vi "Generate_WayPoints_Hopping_CV_VUW.vi"(8 "NumberOfCVsAtEachPoint":i32=1, 11 "Input Cluster":T2={"Scan Rate (um/s)"=15.0, "X Start"=15.0, "X End"=15.0, "Y Start"=15.0, "Y End"=15.0, " Z Start"=15.0, "HoppingDistance"=1.0, "V"=15.0, "Z End"=15.0, "Approach Rate Hopping (um/s)"=15.0, "Retrack Rate (um/s)"=15.0, "V 2"=15.0, "Approach Rate (um/s)"=15.0, "V 3"=15.0, "CV Rate / V/s"=15.0, "V 4"=15.0, "V 1"=15.0, "HoldTime1/s"=15.0, "Hold time 2 / s"=15.0, "Hold time 3/ s"=15.0, "HoppingDistanceBetweenLines"=1.0}) -> (0 "output cluster":T1, 3 "WaitTimeScaler":u64)   [LabVIEW 2023]
uses:
  TypeDefs/WayPointCluster.ctl
  TypeDefsControls/Time.ctl
  User_Vi/Settings.vi
panel:
  in  "WayPointCluster 2":T1
  out "Y  P":dbl
  out "X  P":dbl
  out "HoppingDistanceX":dbl
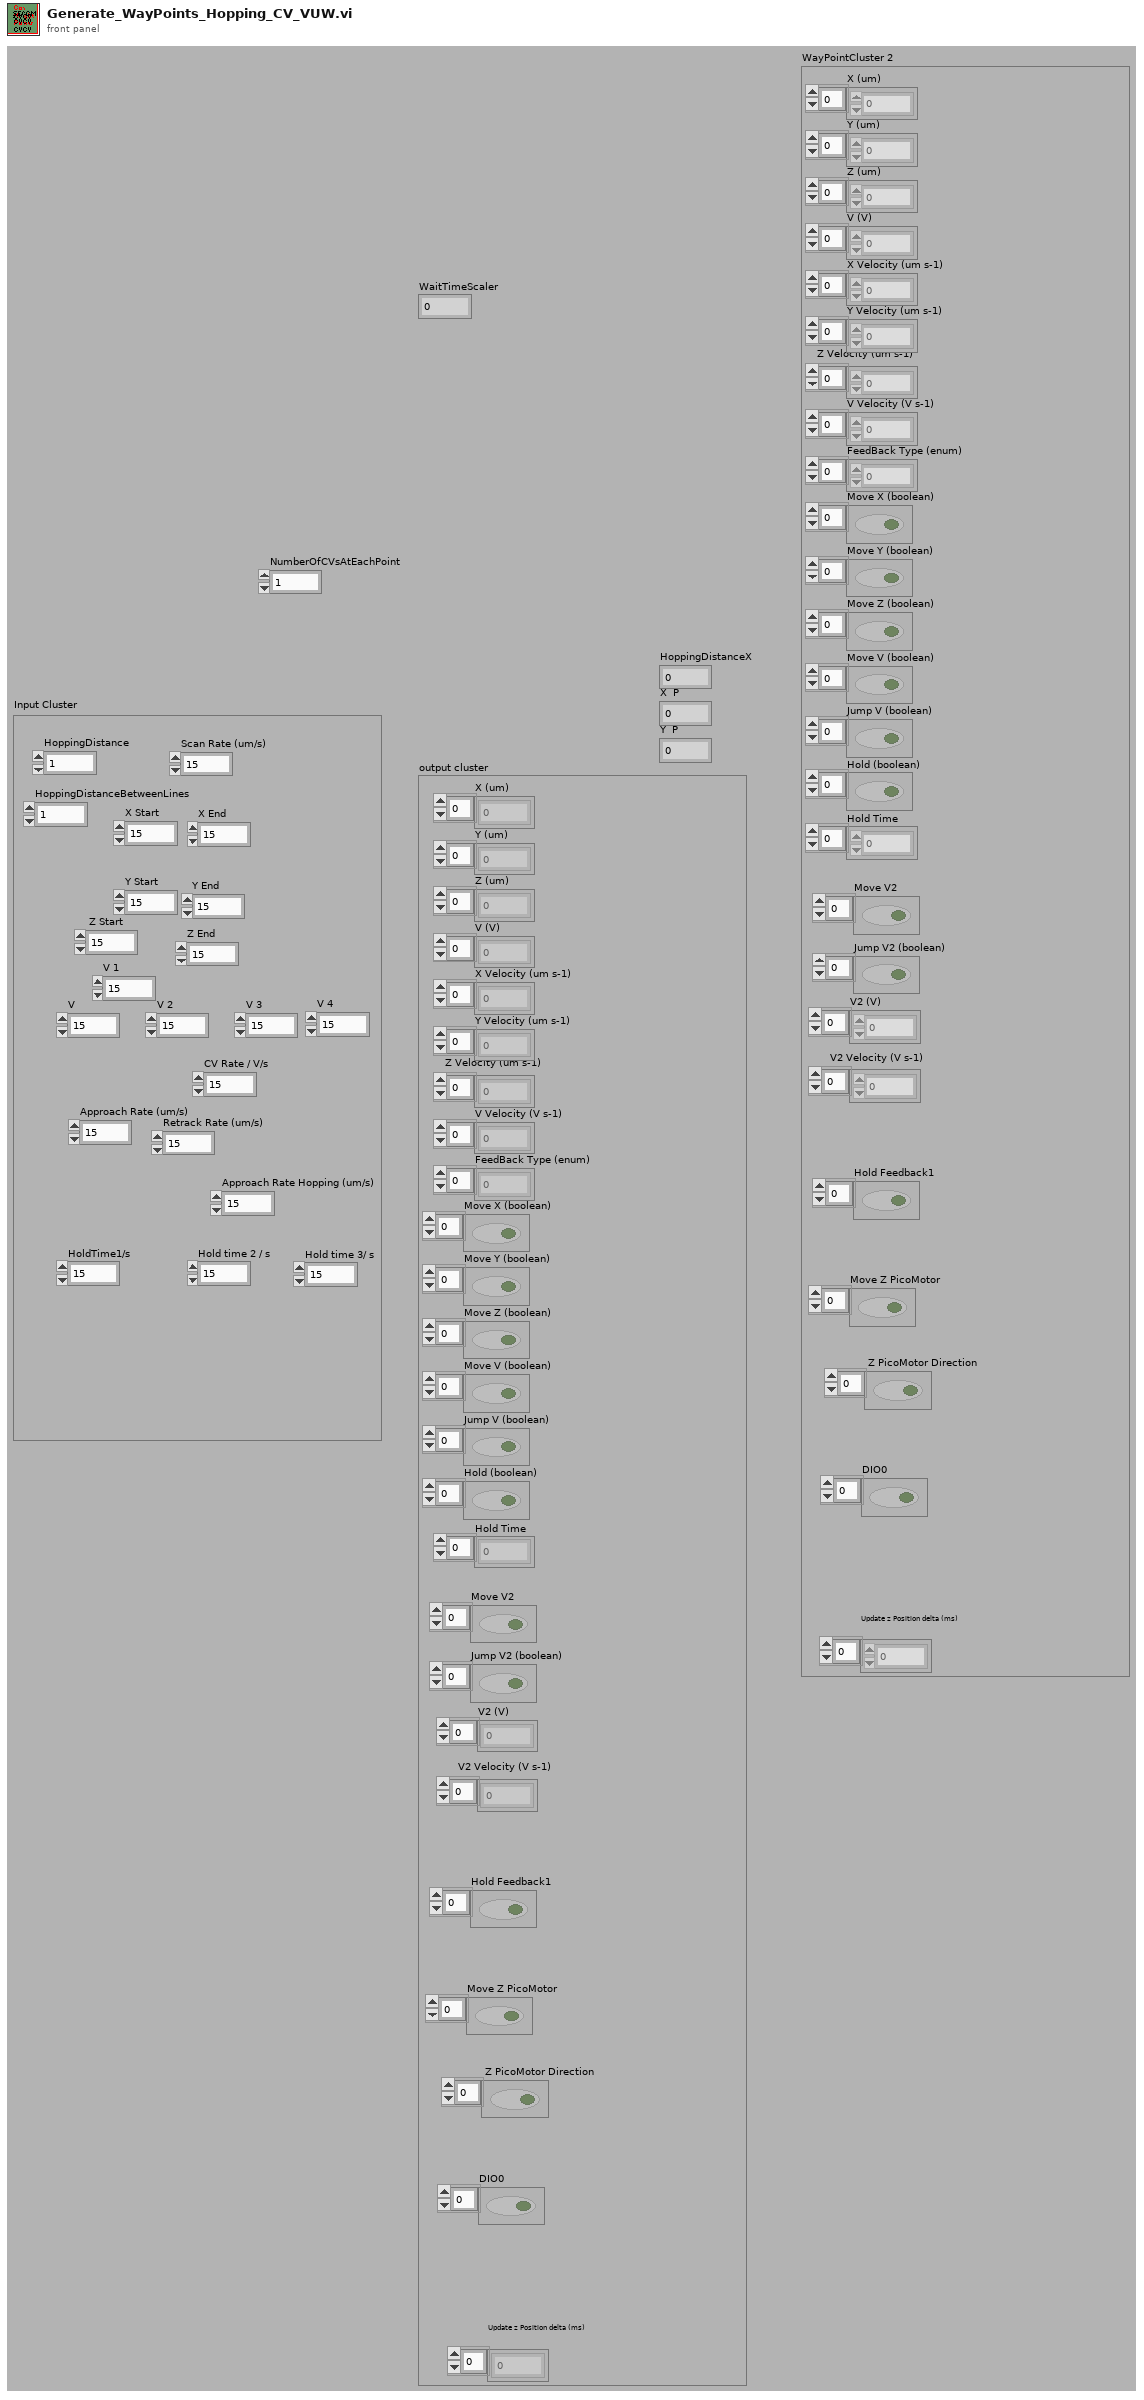
[diagram p1: front panel]
types:
  T1 = typedef "WayPointCluster.ctl" = cluster{"X (um)":dbl[], "Y (um)":dbl[], "Z (um)":dbl[], "V (V)":dbl[], "X Velocity (um s-1)":dbl[], "Y Velocity (um s-1)":dbl[], "Z Velocity (um s-1)":dbl[], "V Velocity (V s-1)":dbl[], "FeedBack Type (enum)":u16[], "Move X (boolean)":bool[], "Move Y (boolean)":bool[], "Move Z (boolean)":bool[], "Move V (boolean)":bool[], "Jump V (boolean)":bool[], "Hold (boolean)":bool[], "Hold Time":u32[], "V2 (V)":dbl[], "Move V2":bool[], "V2 Velocity (V s-1)":dbl[], "Jump V2 (boolean)":bool[], "Update z Position delta (ms)":i16[], "Hold Feedback1":bool[], "Move Z PicoMotor":bool[], " Z PicoMotor Direction":bool[], "DIO0":bool[]}
  T2 = cluster{"Scan Rate (um/s)":dbl, "X Start":dbl, "X End":dbl, "Y Start":dbl, "Y End":dbl, " Z Start":dbl, "HoppingDistance":dbl, "V":dbl, "Z End":dbl, "Approach Rate Hopping (um/s)":dbl, "Retrack Rate (um/s)":dbl, "V 2":dbl, "Approach Rate (um/s)":dbl, "V 3":dbl, "CV Rate / V/s":dbl, "V 4":dbl, "V 1":dbl, "HoldTime1/s":dbl, "Hold time 2 / s":dbl, "Hold time 3/ s":dbl, "HoppingDistanceBetweenLines":dbl}
  T3 = typedef "Time.ctl" = dbl
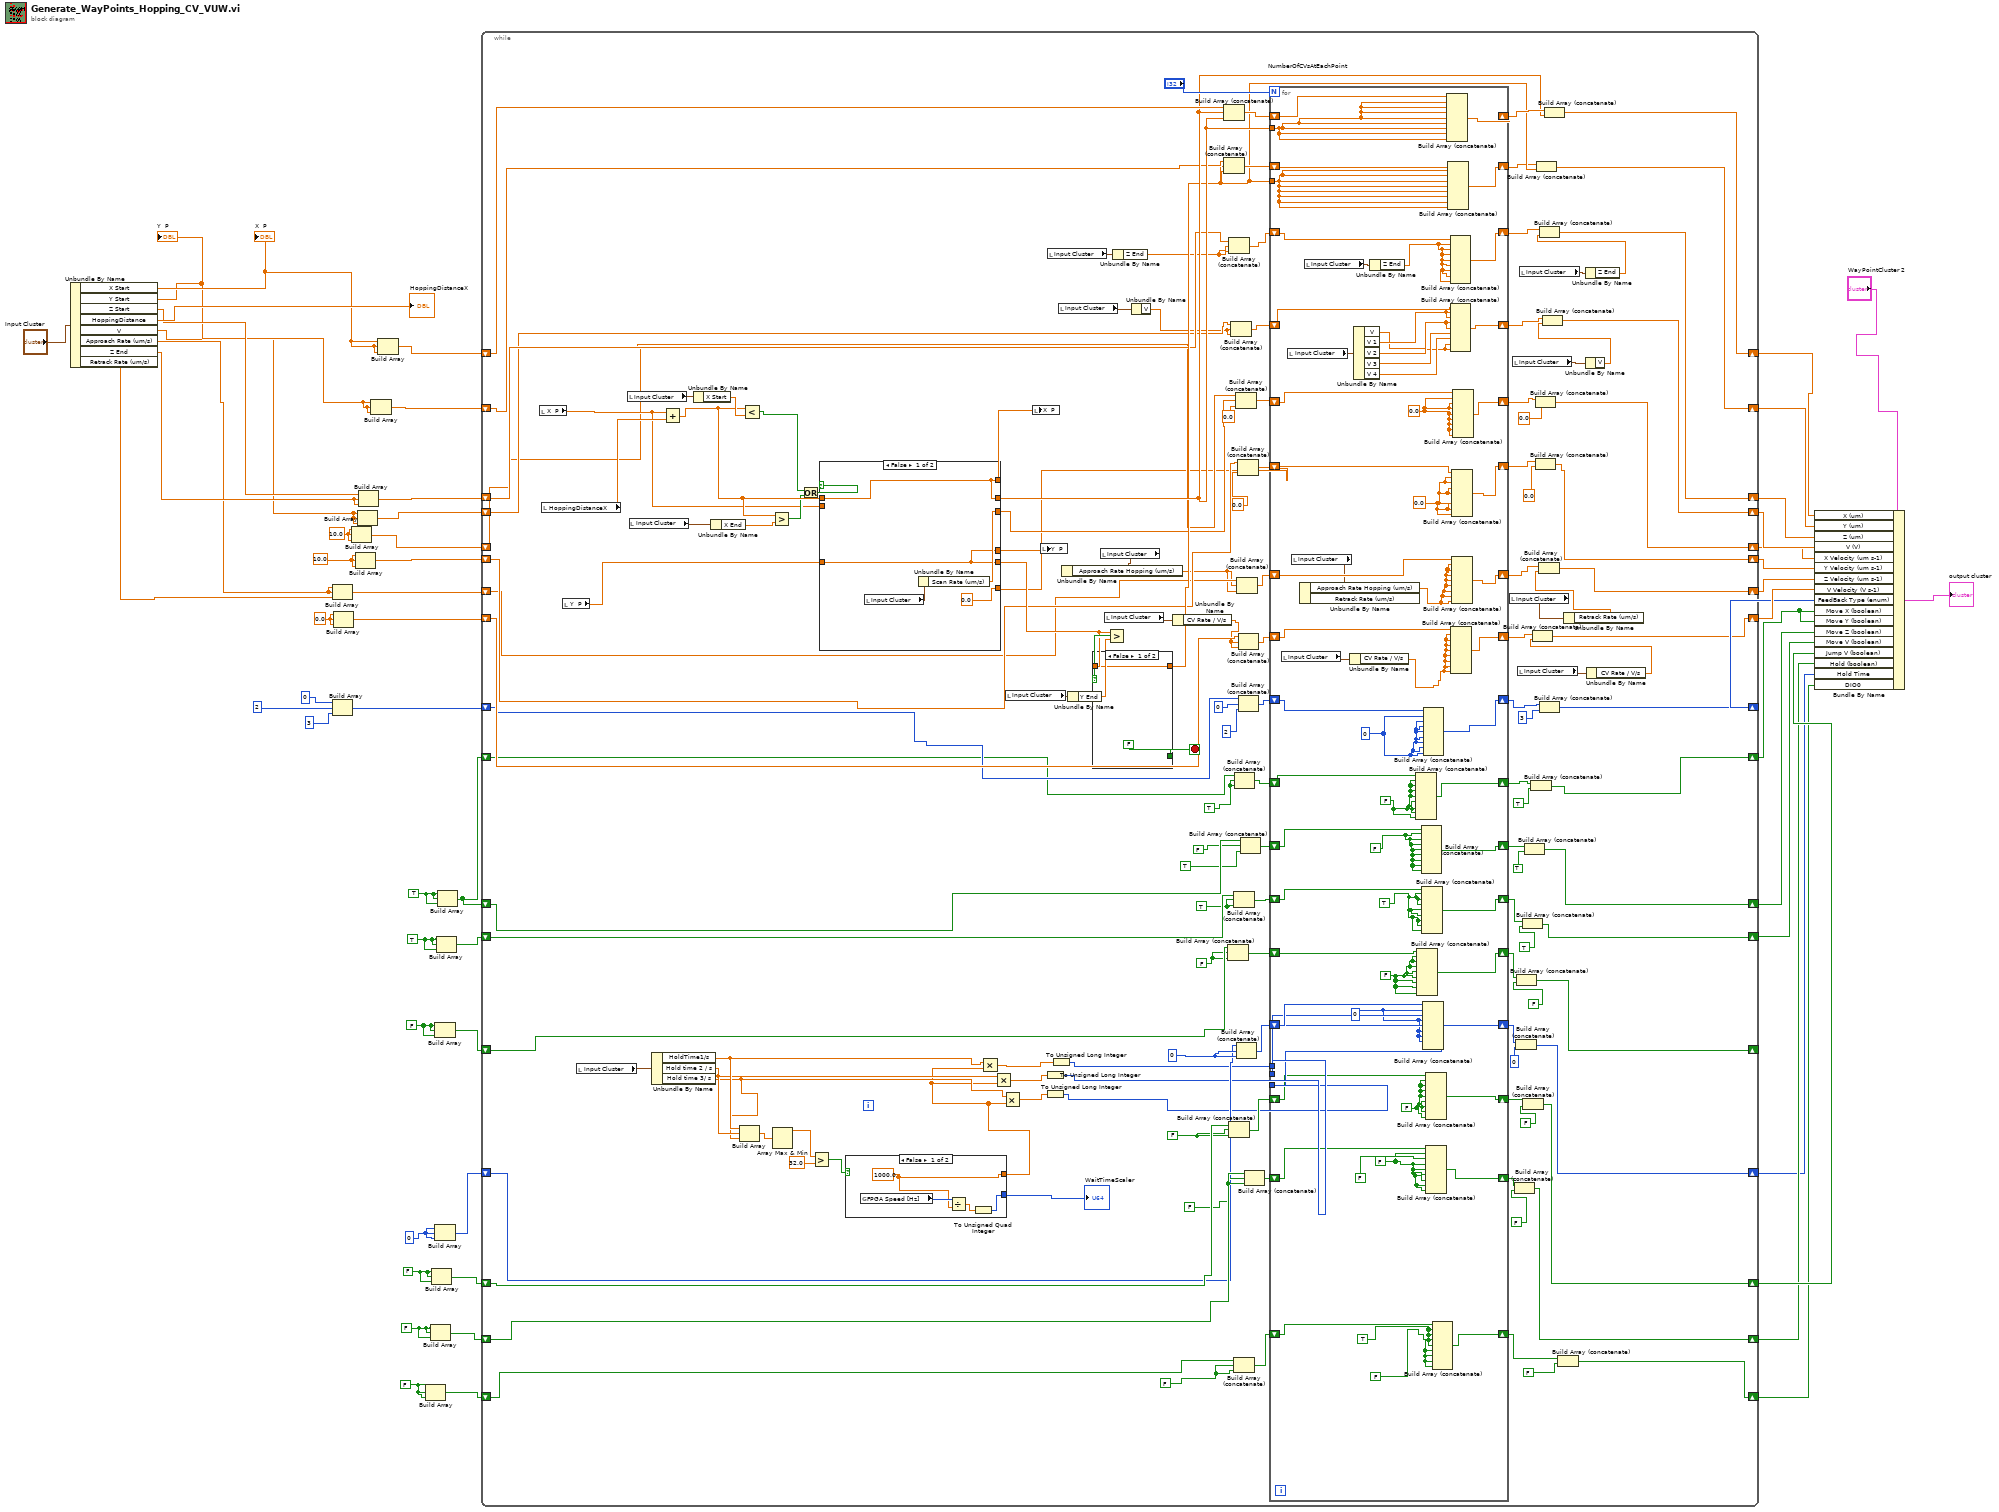
[diagram p0: block diagram]
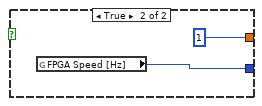
[diagram p2: hidden frame]
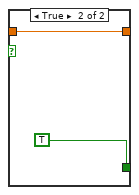
[diagram p3: hidden frame]
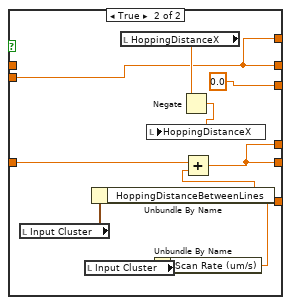
[diagram p4: hidden frame]
diagram:
  w3 = FALSE
  w13 = FALSE
  w21 = FALSE
  w25 = FALSE
  w24 = u32 0 ("element")
  w23 = TRUE
  w19 = TRUE
  w15 = 10.0 ("element")
  w16 = 10.0 ("element")
  w18 = 0.0 ("element")
  n1 = Unbundle By Name("Input Cluster") -> ("X Start"=w37:dbl, "Y Start"=w36:dbl, "Z Start"=w38:dbl, "HoppingDistance"=→"HoppingDistanceX":dbl, "V"=w34:dbl, "Approach Rate (um/s)"=w17:dbl, "Z End"=w35:dbl, "Retrack Rate (um/s)"=w33:dbl)
  "X  P" <- w37
  "Y  P" <- w36
  n2 = Build Array(w17, w17, w33) -> (w45:dbl[])
  n3 = Build Array(u16 0 ("element"), u16 2 ("element"), u16 3 ("element")) -> (w41:u16[])
  n4 = Build Array(w18, w18, w18) -> (w43:dbl[])
  n5 = Build Array(w15, w15, w15) -> (w48:dbl[])
  n6 = Build Array(w16, w16, w16) -> (w47:dbl[])
  n7 = Build Array(w34, w34, w34) -> (w50:dbl[])
  n8 = Build Array(w38, w35, w35) -> (w52:dbl[])
  n9 = Build Array(w36, w36, w36) -> (w53:dbl[])
  n10 = Build Array(w37, w37, w37) -> (w54:dbl[])
  n11 = Build Array(w3, w3, w3) -> (w2:bool[])
  n12 = Build Array(w13, w13, w13) -> (w12:bool[])
  n13 = Build Array(w25, w25, w25) -> (w29:bool[])
  n14 = Build Array(w21, w21, w21) -> (w20:bool[])
  n15 = Build Array(w24, w24, w24) -> (w7:u32[])
  n16 = Build Array(w23, w23, w23) -> (w27:bool[])
  n17 = Build Array(w19, w19, w19) -> (w14:bool[])
  n18 = while {
    shift-right: [w180] -> w9
    shift-left: w54 -> [w183]
    shift-right: [w174] -> w8
    shift-left: w53 -> [w178]
    shift-right: [w168] -> w51
    shift-left: w52 -> [w173]
    shift-right: [w164] -> w49
    shift-left: w50 -> [w162]
    shift-right: [w152] -> w31
    shift-left: w48 -> [w157]
    shift-right: [w144] -> w46
    shift-left: w47 -> [w150]
    shift-right: [w138] -> w44
    shift-left: w45 -> [w143]
    shift-right: [w129] -> w42
    shift-left: w43 -> [w135]
    shift-right: [w123] -> w40
    shift-left: w41 -> [w121]
    shift-right: [w111] -> w30
    shift-left: w14 -> [w114]
    shift-right: [w98] -> _
    shift-left: w20 -> [w101]
    shift-right: [w88] -> w28
    shift-left: w29 -> [w91]
    shift-right: [w104] -> w22
    shift-left: w27 -> [w107]
    shift-right: [w116] -> w10
    shift-left: w14 -> [w120]
    shift-right: [w84] -> w11
    shift-left: w12 -> [w87]
    shift-right: [w72] -> w6
    shift-left: w7 -> [w79]
    shift-right: [w57] -> w1
    shift-left: w2 -> [w62]
    stop <- w191 stop-if-true
    w61 = FALSE
    w81 = FALSE
    w83 = FALSE
    w93 = u32 0 ("element")
    w97 = FALSE
    w102 = TRUE
    w118 = TRUE
    n19 = local read "X  P"() -> (w190:dbl)
    n20 = local read "HoppingDistanceX"() -> (w201:dbl)
    n21 = local read "Y  P"() -> (w189:dbl)
    n22 = local read "Input Cluster"() -> (w185:T2)
    n23 = local read "Input Cluster"() -> (w203:T2)
    n24 = local read "Input Cluster"() -> (w202:T2)
    n25 = Unbundle By Name(w185) -> ("HoldTime1/s"=w71:dbl, "Hold time 2 / s"=w70:dbl, "Hold time 3/ s"=w69:dbl)
    n26 = Add(x=w190, y=w201) -> (x+y=w197:dbl)
    n27 = Unbundle By Name(w203) -> ("X Start"=w200:dbl)
    n28 = Unbundle By Name(w202) -> ("X End"=w198:dbl)
    n29 = Build Array(w71, w70, w69) -> (w68:dbl[])
    n30 = Less?(x=w197, y=w200) -> (x < y?=w199:bool)
    n31 = Greater?(x=w197, y=w198) -> (0:w196:bool)
    n32 = Array Max & Min(array=w68) -> (max value=w66:dbl)  [unwired: 3 out]
    n33 = Or(x=w199, y=w196) -> (x .or. y?=w195:bool)
    n34 = Greater?(x=w66, y=T3 32.0) -> (0:w65:bool)
    n35 = case shown="False" w195 {
      tunnel: w197 -> [w278 _]
      tunnel: [w278 w284] -> w179
      tunnel: w190 -> [_ w284]
      tunnel: w189 -> [w279 w285]
      tunnel: [w279 w283] -> w188
      tunnel: [w281 0.0] -> w155
      tunnel: [0.0 w286] -> w148
      tunnel: [w279 w283] -> w187
      tunnel: [w278 w284] -> w186
      frame False {
        n36 = local read "Input Cluster"() -> (w282:T2)
        n37 = Unbundle By Name(w282) -> ("Scan Rate (um/s)"=w281:dbl)
      }
      frame True {
        n38 = local read "Input Cluster"() -> (w290:T2)
        n39 = local read "Input Cluster"() -> (w288:T2)
        n40 = Unbundle By Name(w290) -> ("HoppingDistanceBetweenLines"=w289:dbl)
        n41 = local read "HoppingDistanceX"() -> (w292:dbl)
        n42 = Unbundle By Name(w288) -> ("Scan Rate (um/s)"=w286:dbl)
        n43 = Negate(x=w292) -> (-x=w291:dbl)
        n44 = local write "HoppingDistanceX"(w291) -> ()
        n45 = Add(x=w285, y=w289) -> (x+y=w283:dbl)
      }
    }
    n46 = case shown="False" w65 {
      tunnel: [w205 w209] -> w64
      tunnel: [w204 1] -> w63
      frame False {
        w204 = 1000.0 ("y")
        n47 = global read "Settings.vi" "FPGA Speed [Hz]"() -> (w207:i64)
        n48 = Divide(x=w207, y=w204) -> (x/y=w206:dbl)
        n49 = To Unsigned Quad Integer(1:w206) -> (0:w205:u64)
      }
      frame True {
        n50 = global read "Settings.vi" "FPGA Speed [Hz]"() -> (w209:i64)
      }
    }
    "WaitTimeScaler" <- w64
    n51 = Multiply(x=w71, y=w63) -> (x*y=w78:dbl)
    n52 = Multiply(x=w70, y=w63) -> (x*y=w76:dbl)
    n53 = Multiply(x=w69, y=w63) -> (x*y=w74:dbl)
    n54 = local read "Input Cluster"() -> (w194:T2)
    n55 = local write "X  P"(w186) -> ()
    n56 = local write "Y  P"(w187) -> ()
    n57 = To Unsigned Long Integer(number=w74) -> (unsigned 32bit integer=w73:u32)
    n58 = To Unsigned Long Integer(number=w76) -> (unsigned 32bit integer=w75:u32)
    n59 = local read "Input Cluster"() -> (w172:T2)
    n60 = To Unsigned Long Integer(number=w78) -> (unsigned 32bit integer=w77:u32)
    n61 = local read "Input Cluster"() -> (w163:T2)
    n62 = Unbundle By Name(w194) -> ("Y End"=w193:dbl)
    n63 = local read "Input Cluster"() -> (w141:T2)
    n64 = Unbundle By Name(w141) -> ("Approach Rate Hopping (um/s)"=w140:dbl)
    n65 = local read "Input Cluster"() -> (w133:T2)
    n66 = Greater?(x=w188, y=w193) -> (0:w192:bool)
    n67 = case shown="False" w192 {
      tunnel: w188 -> [w275 w277]
      tunnel: [w275 w277] -> w176
      tunnel: [FALSE TRUE] -> w191
      frame False {
      }
      frame True {
      }
    }
    n68 = Unbundle By Name(w172) -> ("Z End"=w171:dbl)
    n69 = Unbundle By Name(w163) -> ("V"=w160:dbl)
    n70 = Unbundle By Name(w133) -> ("CV Rate / V/s"=w132:dbl)
    n71 = Build Array (concatenate)(w183, w179, w179) -> (w182:dbl[])
    n72 = Build Array (concatenate)(w178, w176, w176) -> (w177:dbl[])
    n73 = Build Array (concatenate)(w101, w97, w97) -> (w100:bool[])
    n74 = Build Array (concatenate)(w173, w171, w171) -> (w170:dbl[])
    n75 = Build Array (concatenate)(w91, w83, w83) -> (w90:bool[])
    n76 = Build Array (concatenate)(w162, w160, w160) -> (w161:dbl[])
    n77 = Build Array (concatenate)(w107, w102, w102) -> (w106:bool[])
    n78 = Build Array (concatenate)(w62, w61, w61) -> (w60:bool[])
    n79 = Build Array (concatenate)(w120, w118, w118) -> (w119:bool[])
    n80 = Build Array (concatenate)(w157, w155, 0.0 ("element")) -> (w156:dbl[])
    n81 = Build Array (concatenate)(w79, w93, w93) -> (w95:u32[])
    n82 = Build Array (concatenate)(w143, w140, w140) -> (w142:dbl[])
    n83 = Build Array (concatenate)(w150, w148, 0.0 ("element")) -> (w149:dbl[])
    n84 = Build Array (concatenate)(w135, w132, w132) -> (w134:dbl[])
    n85 = Build Array (concatenate)(w121, u16 0 ("element"), u16 2 ("element")) -> (w127:u16[])
    n86 = Build Array (concatenate)(w114, FALSE, TRUE) -> (w113:bool[])
    n87 = Build Array (concatenate)(w87, w81, w81) -> (w86:bool[])
    n88 = for {
      N: "NumberOfCVsAtEachPoint" -> [_]
      shift-right: [w272] -> w181
      shift-left: w182 -> [w273]
      tunnel: w179 -> [w271]
      shift-right: [w268] -> w175
      shift-left: w177 -> [w270]
      tunnel: w176 -> [w269]
      shift-right: [w264] -> w169
      shift-left: w170 -> [w267]
      shift-right: [w262] -> w165
      shift-left: w161 -> [w263]
      shift-right: [w253] -> w153
      shift-left: w156 -> [w255]
      shift-right: [w251] -> w146
      shift-left: w149 -> [w252]
      shift-right: [w248] -> w139
      shift-left: w142 -> [w249]
      shift-right: [w245] -> w130
      shift-left: w134 -> [w244]
      shift-right: [w240] -> w124
      shift-left: w127 -> [w241]
      shift-right: [w237] -> w117
      shift-left: w119 -> [w238]
      shift-right: [w234] -> w112
      shift-left: w113 -> [w235]
      shift-right: [w231] -> w105
      shift-left: w106 -> [w232]
      shift-right: [w228] -> w99
      shift-left: w100 -> [w229]
      shift-right: [w225] -> w94
      shift-left: w95 -> [w226]
      tunnel: w77 -> [w224]
      tunnel: w75 -> [w223]
      tunnel: w73 -> [w221]
      shift-right: [w219] -> w89
      shift-left: w90 -> [w220]
      shift-right: [w217] -> w85
      shift-left: w86 -> [w218]
      shift-right: [w212] -> w59
      shift-left: w60 -> [w213]
      w210 = TRUE
      w211 = FALSE
      w214 = FALSE
      w216 = FALSE
      w222 = u32 0 ("element")
      w227 = FALSE
      w230 = TRUE
      w233 = FALSE
      w236 = FALSE
      w239 = u16 0 ("element")
      w250 = 0.0 ("element")
      w254 = 0.0 ("element")
      n89 = local read "Input Cluster"() -> (w243:T2)
      n90 = local read "Input Cluster"() -> (w261:T2)
      n91 = local read "Input Cluster"() -> (w247:T2)
      n92 = Unbundle By Name(w247) -> ("Approach Rate Hopping (um/s)"=w246:dbl)  [unwired: 1 out]
      n93 = local read "Input Cluster"() -> (w266:T2)
      n94 = Unbundle By Name(w243) -> ("CV Rate / V/s"=w242:dbl)
      n95 = Unbundle By Name(w261) -> ("V"=w256:dbl, "V 1"=w260:dbl, "V 2"=w259:dbl, "V 3"=w258:dbl, "V 4"=w257:dbl)
      n96 = Unbundle By Name(w266) -> ("Z End"=w265:dbl)
      n97 = Build Array (concatenate)(w238, w236, w236, w236, w236, w236, w236, w236, w236) -> (w237:bool[])
      n98 = Build Array (concatenate)(w229, w227, w227, w227, w227, w227, w227, w227, w227) -> (w228:bool[])
      n99 = Build Array (concatenate)(w235, w233, w233, w233, w233, w233, w233, w233, w233) -> (w234:bool[])
      n100 = Build Array (concatenate)(w232, w230, w230, w230, w230, w230, w230, w230, w230) -> (w231:bool[])
      n101 = Build Array (concatenate)(w226, w222, w224, w222, w223, w222, w222, w222, w221) -> (w225:u32[])
      n102 = Build Array (concatenate)(w241, w239, w239, w239, w239, w239, w239, w239, w239) -> (w240:u16[])
      n103 = Build Array (concatenate)(w220, w216, w216, w216, w216, w216, w216, w216, w216) -> (w219:bool[])
      n104 = Build Array (concatenate)(w218, w214, FALSE, w214, w214, w214, w214, w214, w214) -> (w217:bool[])
      n105 = Build Array (concatenate)(w213, w210, w210, w210, w210, w211, w211, w211, w211) -> (w212:bool[])
      n106 = Build Array (concatenate)(w273, w271, w271, w271, w271, w271, w271, w271, w271) -> (w272:dbl[])
      n107 = Build Array (concatenate)(w270, w269, w269, w269, w269, w269, w269, w269, w269) -> (w268:dbl[])
      n108 = Build Array (concatenate)(w267, w265, w265, w265, w265, w265, w265, w265, w265) -> (w264:dbl[])
      n109 = Build Array (concatenate)(w263, w260, w260, w259, w259, w258, w257, w256, w256) -> (w262:dbl[])
      n110 = Build Array (concatenate)(w244, w242, w242, w242, w242, w242, w242, w242, w242) -> (w245:dbl[])
      n111 = Build Array (concatenate)(w252, w250, w250, w250, w250, w250, w250, w250, w250) -> (w251:dbl[])
      n112 = Build Array (concatenate)(w249, w246, w246, w246, w246, w246, w246, w246, w246) -> (w248:dbl[])
      n113 = Build Array (concatenate)(w255, w254, w254, w254, w254, w254, w254, w254, w254) -> (w253:dbl[])
    }
    n114 = local read "Input Cluster"() -> (w137:T2)
    n115 = local read "Input Cluster"() -> (w159:T2)
    n116 = Build Array (concatenate)(w85, FALSE) -> (w84:bool[])
    n117 = Build Array (concatenate)(w94, u32 0 ("element")) -> (w72:u32[])
    n118 = Build Array (concatenate)(w99, FALSE) -> (w98:bool[])
    n119 = local read "Input Cluster"() -> (w131:T2)
    n120 = local read "Input Cluster"() -> (w167:T2)
    n121 = Build Array (concatenate)(w105, TRUE) -> (w104:bool[])
    n122 = Build Array (concatenate)(w89, FALSE) -> (w88:bool[])
    n123 = Build Array (concatenate)(w112, TRUE) -> (w111:bool[])
    n124 = Build Array (concatenate)(w117, TRUE) -> (w116:bool[])
    n125 = Build Array (concatenate)(w153, 0.0 ("element")) -> (w152:dbl[])
    n126 = Build Array (concatenate)(w146, 0.0 ("element")) -> (w144:dbl[])
    n127 = Build Array (concatenate)(w175, w176) -> (w174:dbl[])
    n128 = Build Array (concatenate)(w124, u16 3 ("element")) -> (w123:u16[])
    n129 = Build Array (concatenate)(w181, w179) -> (w180:dbl[])
    n130 = Build Array (concatenate)(w59, FALSE) -> (w57:bool[])
    n131 = Unbundle By Name(w137) -> ("Retrack Rate (um/s)"=w136:dbl)
    n132 = Build Array (concatenate)(w139, w136) -> (w138:dbl[])
    n133 = Unbundle By Name(w167) -> ("Z End"=w166:dbl)
    n134 = Build Array (concatenate)(w169, w166) -> (w168:dbl[])
    n135 = Unbundle By Name(w159) -> ("V"=w158:dbl)
    n136 = Build Array (concatenate)(w165, w158) -> (w164:dbl[])
    n137 = Unbundle By Name(w131) -> ("CV Rate / V/s"=w128:dbl)
    n138 = Build Array (concatenate)(w130, w128) -> (w129:dbl[])
  }
  n139 = Bundle By Name(cluster="WayPointCluster 2", "X (um)"=w9, "Y (um)"=w8, "Z (um)"=w51, "V (V)"=w49, "X Velocity (um s-1)"=w31, "Y Velocity (um s-1)"=w46, "Z Velocity (um s-1)"=w44, "V Velocity (V s-1)"=w42, "FeedBack Type (enum)"=w40, "Move X (boolean)"=w10, "Move Y (boolean)"=w10, "Move Z (boolean)"=w30, "Move V (boolean)"=w22, "Jump V (boolean)"=w28, "Hold (boolean)"=w11, "Hold Time"=w6, "DIO0"=w1) -> (→"output cluster":T1)
